vi "Parse GSV Satellite.vi"(8 "Message SV Num":i32, 9 "Message Num":i32, 11 "Fields In":string[](array[string])) -> (0 "SNR":i32, 1 "Azimuth":i32, 2 "Elevation":i32, 3 "Fields":string[](array[string]), 5 "Channel":i32, 7 "PRN":i32)   [LabVIEW 2020, in "nmea.lvlib" / "nmea.lvclass"]
uses:
  nmea.lvclass
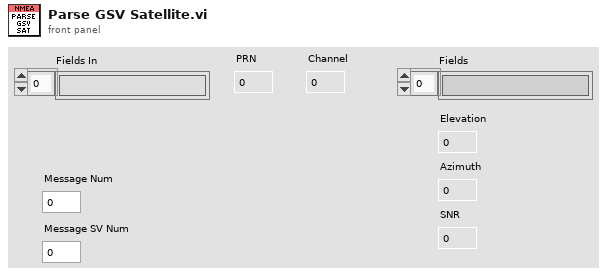
[diagram p1: front panel]
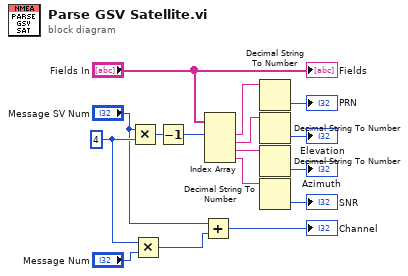
[diagram p0: block diagram]
diagram:
  w13 = 4 ("y")
  n1 = Multiply(x="Message SV Num", y=w13) -> (x*y=w16:i32)
  n2 = Multiply(x=w13, y="Message Num") -> (x*y=w12:i32)
  n3 = Decrement(x=w16) -> (x-1=w1:i32)
  n4 = Add(x="Message SV Num", y=w12) -> (x+y=→"Channel":i32)
  n5 = Index Array(array="Fields In", index #1=w1) -> (element #1=w8:string, element #2=w9:string, element #3=w7:string, element #4=w6:string)  [unwired: 3 in]
  n6 = Decimal String To Number(string=w8) -> (number=→"PRN":i32)  [unwired: 2 in, 1 out]
  n7 = Decimal String To Number(string=w9) -> (number=→"Elevation":i32)  [unwired: 2 in, 1 out]
  n8 = Decimal String To Number(string=w7) -> (number=→"Azimuth":i32)  [unwired: 2 in, 1 out]
  n9 = Decimal String To Number(string=w6) -> (number=→"SNR":i32)  [unwired: 2 in, 1 out]
  "Fields" <- "Fields In"
